vi "GenerateProjectDocumentation.vi"(8 "error in":errorcluster) -> (0 "error out":errorcluster)   [LabVIEW 2020, in "CICD.lvlib"]
uses:
  CICD.lvlib
  <vilib>/Wiresmith Technology/G CLI/Argument Parser/Option Class/Option Configuration.ctl
  <vilib>/Wiresmith Technology/G CLI/Argument Parser/Option Class/Argument Type.ctl
  Helpers/AntidocArgs2--cluster.ctl
  <vilib>/Wiresmith Technology/G CLI/CLI Class/CLI.lvclass
  <vilib>/Wiresmith Technology/G CLI/Argument Parser/Option Set Class/Option Set.lvclass
  <vilib>/Wiresmith Technology/G CLI/Argument Parser/Option Class/Option.lvclass
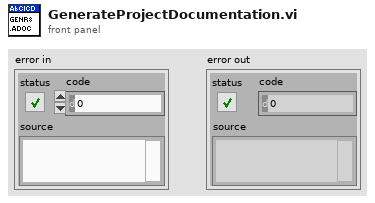
[diagram p1: front panel]
types:
  T1 = typedef "Option Parser.lvlib/Option.lvclass/Option Configuration.ctl" = cluster{"Option Type":T2, "Option Labels":string[], "Key":string, "Description":string, "Required":bool, "Default Value":string}
  T2 = typedef "Option Parser.lvlib/Option.lvclass/Argument Type.ctl" = enum16{"flag", "value"}
  T3 = typedef "CICD.lvlib/AntidocArgs2--cluster.ctl" = cluster{"ProjectPath":path, "ReportDir":path, "ReportFile":string, "ReportTitle":string, "ReportAuthor":string, "Commit":string, "Date":string, "Tag":string}
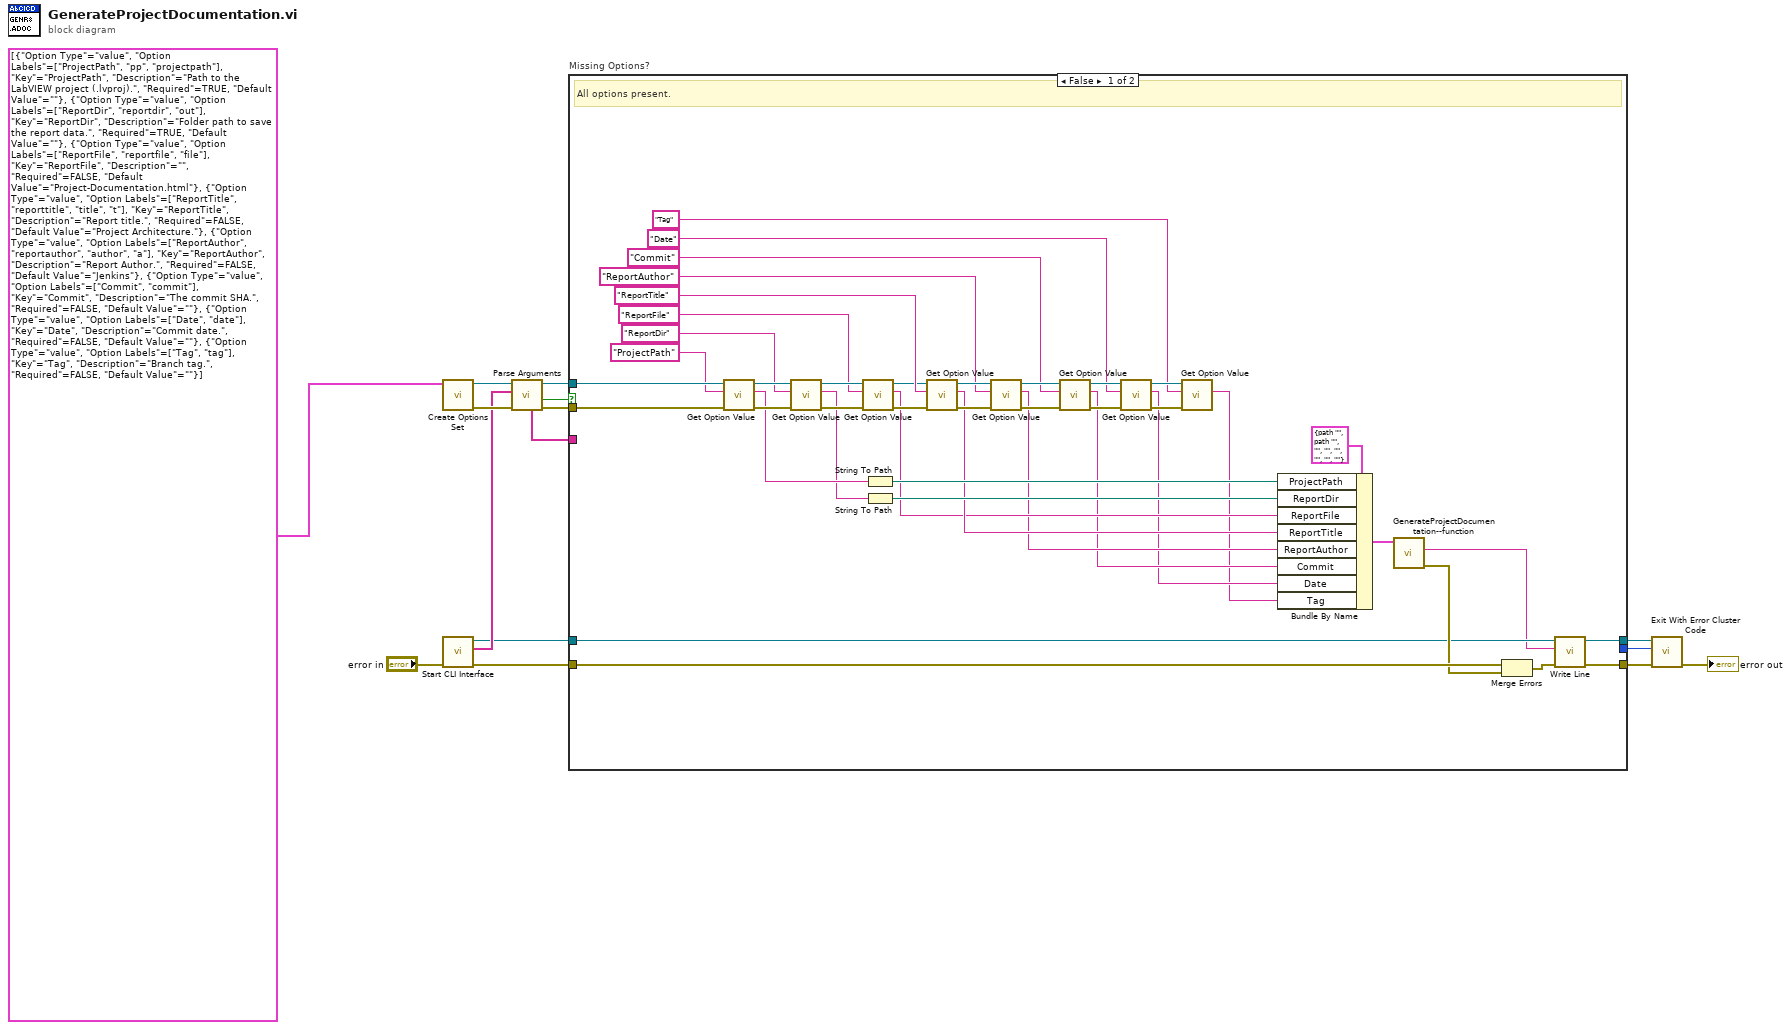
[diagram p0: block diagram]
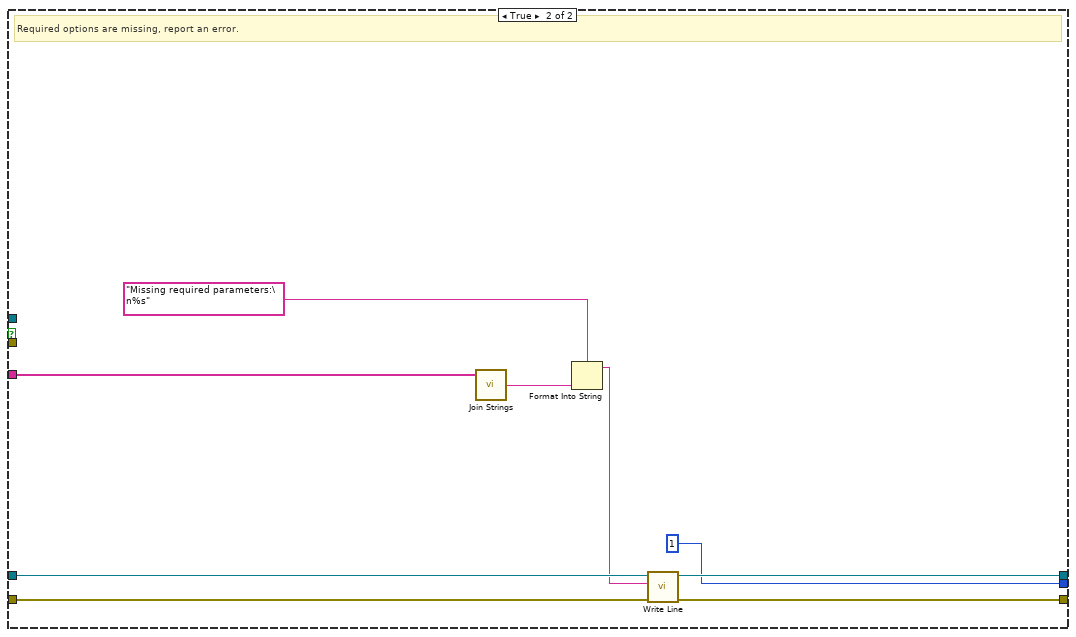
[diagram p2: hidden frame]
diagram:
  n1 = call <vilib>:"Create Options Set.vi"("Options"=T1[] [{"Option Type"=enum."value", "Option Labels"=["ProjectPath", "pp", "projectpath"], "Key"="ProjectPath", "Description"="Path to the LabVIEW project (.lvproj).", "Required"=TRUE, "Default Value"=""}, {"Option Type"=enum."value", "Option Labels"=["ReportDir", "reportdir", "out"], "Key"="ReportDir", "Description"="Folder path to save the report data.", "Required"=TRUE, "Default Value"=""}, {"Option Type"=enum."value", "Option Labels"=["ReportFile", "reportfile", "file"], "Key"="ReportFile", "Description"="", "Required"=FALSE, "Default Value"="Project-Documentation.html"}, {"Option Type"=enum."value", "Option Labels"=["ReportTitle", "reporttitle", "title", "t"], "Key"="ReportTitle", "Description"="Report title.", "Required"=FALSE, "Default Value"="Project Architecture."}, {"Option Type"=enum."value", "Option Labels"=["ReportAuthor", "reportauthor", "author", "a"], "Key"="ReportAuthor", "Description"="Report Author.", "Required"=FALSE, "Default Value"="Jenkins"}, {"Option Type"=enum."value", "Option Labels"=["Commit", "commit"], "Key"="Commit", "Description"="The commit SHA.", "Required"=FALSE, "Default Value"=""}, {"Option Type"=enum."value", "Option Labels"=["Date", "date"], "Key"="Date", "Description"="Commit date.", "Required"=FALSE, "Default Value"=""}, {"Option Type"=enum."value", "Option Labels"=["Tag", "tag"], "Key"="Tag", "Description"="Branch tag.", "Required"=FALSE, "Default Value"=""}]) -> ("error out"=w14:errorcluster, "Option Set out"=w9:refnum<class "Option Set.lvclass">)  [unwired: 9 in]
  n2 = call <vilib>:"Start CLI Interface.vi"("error in (no error)"="error in") -> ("error out"=w12:errorcluster, "Custom Parameters"=w8:string[], "CLI out"=w5:refnum<class "CLI.lvclass">)  [unwired: 7 in, 1 out]
  n3 = call <vilib>:"Parse Arguments.vi"("error in (no error)"=w14, "Arguments"=w8, "Option Set in"=w9) -> ("error out"=w13:errorcluster, "Missing Options"=w7:bool, "Option Set out"=w2:refnum<class "Option Set.lvclass">, "Missing Option Keys"=w6:string[])  [unwired: 5 in]
  n4 = case "Missing Options?" shown="False" w7 {
    tunnel: w13 -> [w57 _]
    tunnel: w6 -> [_ w63]
    tunnel: w12 -> [w58 w67]
    tunnel: w5 -> [w46 w62]
    tunnel: [w56 w66] -> w11
    tunnel: [w45 w60] -> w4
    tunnel: [_ 1 ("No Error Code (0)")] -> w3
    tunnel: w2 -> [w44 _]
    frame False {
      # "All options present."
      n5 = call <vilib>:"Get Option Value.vi"("error in (no error)"=w57, "Option Key"="ProjectPath" ("Key"), "Option Set in"=w44) -> ("error out"=w55:errorcluster, "Value"=w27:string, "Option Set out"=w43:refnum<class "Option Set.lvclass">)  [unwired: 5 in, 1 out]
      n6 = call <vilib>:"Get Option Value.vi"("error in (no error)"=w55, "Option Key"="ReportDir" ("Key"), "Option Set in"=w43) -> ("error out"=w53:errorcluster, "Value"=w25:string, "Option Set out"=w36:refnum<class "Option Set.lvclass">)  [unwired: 5 in, 1 out]
      n7 = call <vilib>:"Get Option Value.vi"("error in (no error)"=w53, "Option Key"="ReportFile" ("Key"), "Option Set in"=w36) -> ("error out"=w51:errorcluster, "Value"=w22:string, "Option Set out"=w35:refnum<class "Option Set.lvclass">)  [unwired: 5 in, 1 out]
      n8 = String To Path(string=w27) -> (path=w26:path)
      n9 = String To Path(string=w25) -> (path=w24:path)
      n10 = call <vilib>:"Get Option Value.vi"("error in (no error)"=w51, "Option Key"="ReportTitle" ("Key"), "Option Set in"=w35) -> ("error out"=w54:errorcluster, "Value"=w23:string, "Option Set out"=w42:refnum<class "Option Set.lvclass">)  [unwired: 5 in, 1 out]
      n11 = call <vilib>:"Get Option Value.vi"("error in (no error)"=w54, "Option Key"="ReportAuthor" ("Key"), "Option Set in"=w42) -> ("error out"=w52:errorcluster, "Value"=w21:string, "Option Set out"=w41:refnum<class "Option Set.lvclass">)  [unwired: 5 in, 1 out]
      n12 = call <vilib>:"Get Option Value.vi"("error in (no error)"=w52, "Option Key"="Commit" ("Key"), "Option Set in"=w41) -> ("error out"=w50:errorcluster, "Value"=w20:string, "Option Set out"=w33:refnum<class "Option Set.lvclass">)  [unwired: 5 in, 1 out]
      n13 = call <vilib>:"Get Option Value.vi"("error in (no error)"=w50, "Option Key"="Date" ("Key"), "Option Set in"=w33) -> ("error out"=w49:errorcluster, "Value"=w19:string, "Option Set out"=w32:refnum<class "Option Set.lvclass">)  [unwired: 5 in, 1 out]
      n14 = call <vilib>:"Get Option Value.vi"("error in (no error)"=w49, "Option Key"="Tag" ("Key"), "Option Set in"=w32) -> ("Value"=w18:string)  [unwired: 5 in, 3 out]
      n15 = Bundle By Name(cluster=T3 {"ProjectPath"=path "", "ReportDir"=path "", "ReportFile"="", "ReportTitle"="", "ReportAuthor"="", "Commit"="", "Date"="", "Tag"=""} ("Antidoc Args"), "ProjectPath"=w26, "ReportDir"=w24, "ReportFile"=w22, "ReportTitle"=w23, "ReportAuthor"=w21, "Commit"=w20, "Date"=w19, "Tag"=w18) -> (w17:T3)
      n16 = call "GenerateProjectDocumentation--function.vi"("Antidoc Args"=w17) -> ("error out"=w47:errorcluster, "Generation Details"=w16:string)  [unwired: 8 in, 1 out]
      n17 = Merge Errors(w58, w47) -> (w48:errorcluster)
      n18 = call <vilib>:"Write Line.vi"("error in (no error)"=w48, "Text to Write"=w16, "CLI in"=w46) -> ("error out"=w56:errorcluster, "CLI out"=w45:refnum<class "CLI.lvclass">)  [unwired: 7 in]
    }
    frame True {
      # "Required options are missing, report an error."
      n19 = call <vilib>:"Join Strings.vi"("Strings In"=w63) -> ("String"=w64:string)  [unwired: 2 in]
      n20 = Format Into String(format string="Missing required parameters:\n%s" ("Text to Write"), w64) -> (resulting string=w61:string)  [unwired: 2 in, 1 out]
      n21 = call <vilib>:"Write Line.vi"("error in (no error)"=w67, "Text to Write"=w61, "CLI in"=w62) -> ("error out"=w66:errorcluster, "CLI out"=w60:refnum<class "CLI.lvclass">)  [unwired: 7 in]
    }
  }
  n22 = call <vilib>:"Exit With Error Cluster Code.vi"("error in (no error)"=w11, "No Error Code (0)"=w3, "CLI in"=w4) -> ("error out"=→"error out":errorcluster)  [unwired: 8 in]
